vi "mod_GSM Differentiate Bits.vi"(1 "bits in":i8[](array[numeric]), 2 "initial bit":i8) -> (0 "diffed bits":i8[](array[numeric]))   [LabVIEW 2020, in "niDMT.lvlib"]
uses:
  <vilib>/addons/Modulation/niDMT.lvlib
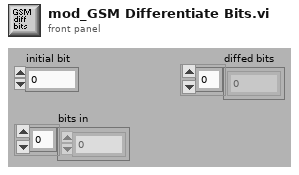
[diagram p1: front panel]
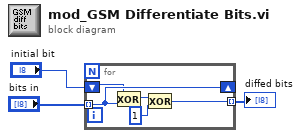
[diagram p0: block diagram]
diagram:
  n1 = for {
    tunnel: "bits in" -> [w8] mode=indexing
    tunnel: [w5] -> w3 mode=indexing
    shift-right: [w8] -> _
    shift-left: "initial bit" -> [w7]
    n2 = Exclusive Or(1:w8, 2:w7) -> (0:w6:i8)
    n3 = Exclusive Or(1:i8 1 ("y"), 2:w6) -> (0:w5:i8)
  }
  "diffed bits" <- w3
